vi "OctaveBandAnalysis.vi"(2 "Filter":T1 items=["None", "1 Octave", "1/3 Octave", "1/12 Octave", "Custom"], 3 "Current FRF":cluster{dbl, "df":dbl, dbl[]}(graph)={0.0, "df"=1.160997732426306, array[22050 elements]}) -> (1 "FRF Bands 2":cluster{"Fctr":ext[], "magnitude":dbl[]}[](graph)=[{"Fctr"=[25.73721928961165, 32.352028870043036, 40.66693298256041, 51.11887865986131, 64.25711416600414, 80.77205191484325, 101.53154954452943, 127.62651571339914, 160.428237195363, 201.66043980553155, 253.48986994750726, 318.6401568298155, 400.534938794811, 503.47777502835936, 632.87829698514, 795.5364837549187, 1000.0, 1257.0133745218284, 1580.0826237267545, 1986.1849908740721, 2496.6610978032245, 3138.3363915870036, 3944.9308179734376, 4958.830799755948, 6233.3166372840005, 7835.362380695417, 9849.155306759334, 12380.519948339124, 15562.479158596574, 19562.244443073105], "magnitude"=[-59.22433454414856, -66.2314935000544, -66.10124910819798, -73.25405372586764, -72.91725269257354, -79.52986667892496, -79.44581491850705, -83.20512373119247, -82.7593394941647, -89.63537694174055, -87.7998305536222, -89.44346376976519, -90.85831760499235, -98.17900781672215, -88.73245480537615, -88.59138292453578, -92.70765312280365, -94.03489436301587, -92.74361707931767, -94.5497480805882, -97.3842899584312, -97.20730378363506, -99.43262058496059, -102.03224809586673, -105.2012624044125, -106.33142078355012, -106.10469195235223, -106.06589607465796, -106.30619707837911, -106.64145916286945]}, {"Fctr"=array[22050 elements], "magnitude"=array[22050 elements]}])   [LabVIEW 2014]
uses:
  <userlib>/CurtinCode/FilterCtrl.ctl
  <vilib>/Analysis/baseanly.llb/Mean (DBL).vi
  <vilib>/Analysis/NI_AALBase.lvlib
panel:
  out "FRF Bands":cluster{"Fctr":ext[], dbl[]}(graph)
  out "Fmax":ext[](array[numeric])=[28.85569721029358, 36.271997324491245, 45.594385757505464, 57.312752700291945, 72.04289667492901, 90.55888465967992, 113.83372919899729, 143.09052007483558, 179.8666975013525, 226.09484439027202, 284.2042433090035, 357.24853493527326, 449.0661864419671, 564.4822024030656, 709.5616781001912, 891.9285194200927, 1121.1660780285088, 1409.3207551420194, 1771.5350382047216, 2226.843236457373, 2799.1717311903926, 3518.5963036897433, 4422.922613281076, 5559.67287936935, 6988.583167333556, 8784.7425102964, 11042.538827173037, 13880.618994433093, 17448.12372264413, 21932.524879675264]
  out "Fmin":ext[](array[numeric])=[22.955759894973568, 28.855697210293577, 36.27199732449124, 45.59438575750547, 57.31275270029194, 72.042896674929, 90.55888465967992, 113.83372919899729, 143.09052007483558, 179.8666975013525, 226.094844390272, 284.20424330900346, 357.2485349352732, 449.0661864419671, 564.4822024030656, 709.5616781001912, 891.9285194200927, 1121.1660780285088, 1409.3207551420196, 1771.5350382047213, 2226.843236457373, 2799.171731190392, 3518.5963036897433, 4422.922613281076, 5559.672879369349, 6988.583167333556, 8784.7425102964, 11042.538827173037, 13880.61899443309, 17448.12372264413]
  out "Fctr":ext[](array[numeric])=[25.73721928961165, 32.352028870043036, 40.66693298256041, 51.11887865986131, 64.25711416600414, 80.77205191484325, 101.53154954452943, 127.62651571339914, 160.428237195363, 201.66043980553155, 253.48986994750726, 318.6401568298155, 400.534938794811, 503.47777502835936, 632.87829698514, 795.5364837549187, 1000.0, 1257.0133745218284, 1580.0826237267545, 1986.1849908740721, 2496.6610978032245, 3138.3363915870036, 3944.9308179734376, 4958.830799755948, 6233.3166372840005, 7835.362380695417, 9849.155306759334, 12380.519948339124, 15562.479158596574, 19562.244443073105]
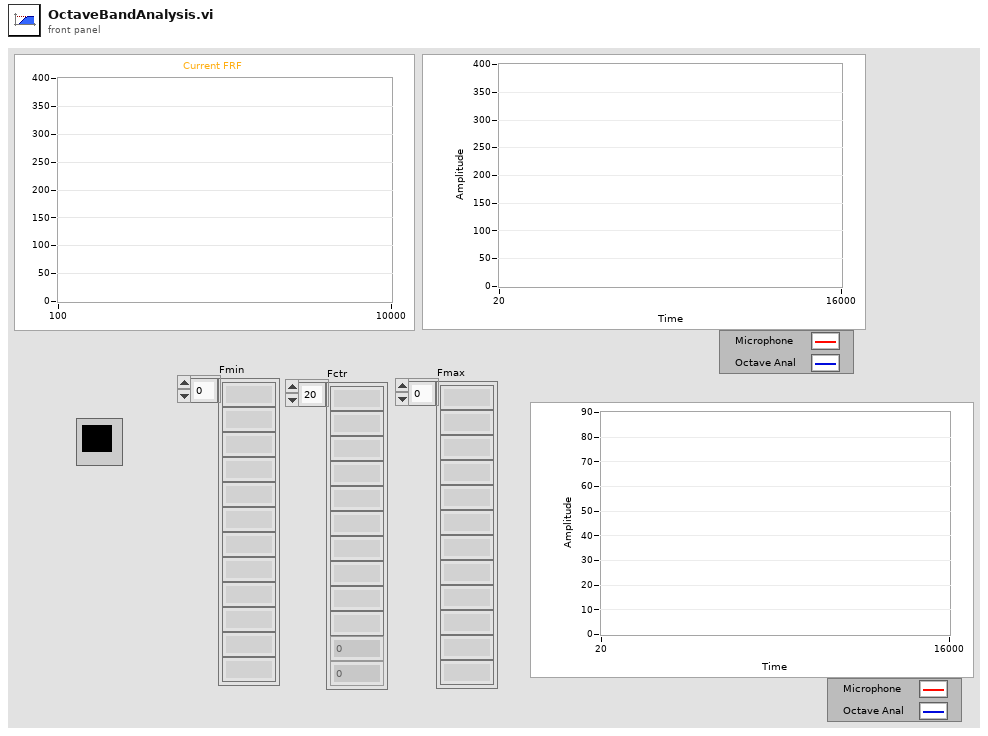
[diagram p1: front panel]
types:
  T1 = typedef "FilterCtrl.ctl" = i8
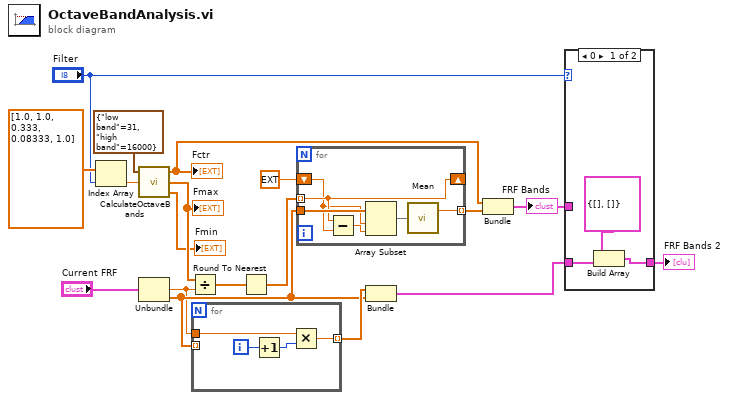
[diagram p0: block diagram]
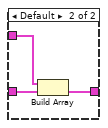
[diagram p2: hidden frame]
diagram:
  n1 = Index Array(array=dbl[] [1.0, 1.0, 0.333, 0.08333, 1.0], index="Filter") -> (element=w2:dbl)
  n2 = call <userlib>:"CalculateOctaveBands.vi"("Octave"=w2, "frequency range"=cluster{"low band":u16, "high band":u16} {"low band"=31, "high band"=16000}) -> ("Fmin"=→"Fmin":ext[], "Fmax"=w12:ext[], "Fctr"=w15:ext[])  [unwired: 1 in]
  "Fctr" <- w15
  "Fmax" <- w12
  n3 = Unbundle("Current FRF") -> ("df"=w9:dbl, w10:dbl[])  [unwired: 1 out]
  n4 = Divide(x=w12, y=w9) -> (x/y=w18:ext[])
  n5 = for {
    tunnel: w10 -> [_] mode=indexing
    tunnel: w9 -> [w21]
    tunnel: [w19] -> w13 mode=indexing
    i -> [w22]
    n6 = Increment(x=w22) -> (x+1=w20:i32)
    n7 = Multiply(x=w21, y=w20) -> (x*y=w19:dbl)
  }
  n8 = Round To Nearest(number=w18) -> (nearest integer value=w17:ext[])
  n9 = for {
    tunnel: w10 -> [w28]
    shift-right: [w27] -> _
    shift-left: ext 0.0 -> [w25]
    tunnel: w17 -> [w27] mode=indexing
    tunnel: [w23] -> w14 mode=indexing
    n10 = Subtract(x=w27, y=w25) -> (x-y=w26:ext)
    n11 = Array Subset(array=w28, index=w25, length=w26) -> (w24:dbl[])
    n12 = call-poly <vilib>:"Mean.vi"("X"=w24) -> ("mean"=w23:dbl)  [unwired: 1 out]
  }
  n13 = Bundle(w13, w10) -> (w7:cluster{dbl[], dbl[]})  [unwired: 1 in]
  n14 = Bundle("Fctr"=w15, w14) -> (w6:cluster{"Fctr":ext[], dbl[]})  [unwired: 1 in]
  "FRF Bands" <- w6
  n15 = case shown="0" "Filter" {
    tunnel: [w30 w34] -> w8
    tunnel: w7 -> [w31 w33]
    tunnel: w6 -> [_ w32]
    frame 0 {
      n16 = Build Array(cluster{dbl[], dbl[]} {[], []} ("output cluster"), w31) -> (w30:cluster{dbl[], dbl[]}[])
    }
    frame Default {
      n17 = Build Array(w32, w33) -> (w34:cluster{"Fctr":ext[], dbl[]}[])
    }
  }
  "FRF Bands 2" <- w8
